vi "Rename Link.vi"(8 "error in (no error)":errorcluster, 9 "New Name":string, 10 "Old Name":string, 11 "Termination in":refnum<class "Termination.lvclass">) -> (0 "error out":errorcluster, 3 "Termination out":refnum<class "Termination.lvclass">)   [LabVIEW 2015, in "Termination.lvclass"]
uses:
  Termination.lvclass
  Termination.lvclass/Termination.ctl
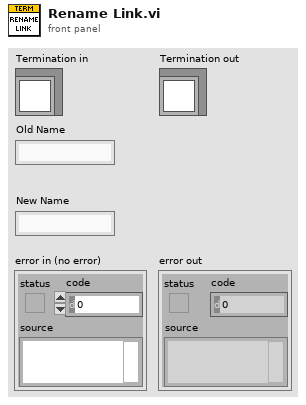
[diagram p1: front panel]
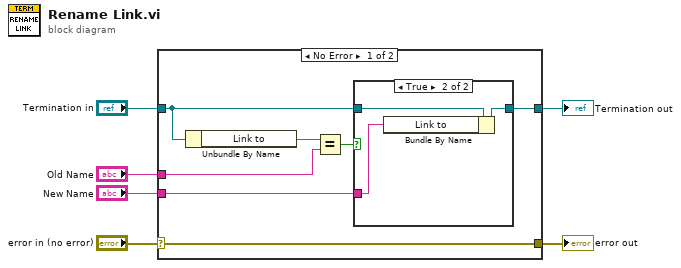
[diagram p0: block diagram]
diagram:
  n1 = case shown="No Error" "error in (no error)" {
    selector: "error in (no error)" -> [w13 w19]
    tunnel: [w13 w19] -> w5
    tunnel: [w9 w18] -> w3
    tunnel: "Termination in" -> [w10 w18]
    tunnel: "Old Name" -> [w11 _]
    tunnel: "New Name" -> [w7 _]
    frame No Error {
      n2 = Unbundle By Name(w10) -> ("Link to"=w12:string)
      n3 = Equal?(x=w12, y=w11) -> (x = y?=w8:bool)
      n4 = case shown="True" w8 {
        tunnel: w10 -> [w14 w17]
        tunnel: [w14 w16] -> w9
        tunnel: w7 -> [_ w15]
        frame False {
        }
        frame True {
          n5 = Bundle By Name(cluster=w17, "Link to"=w15) -> (w16:refnum<class "Termination.lvclass">)
        }
      }
    }
    frame Error {
    }
  }
  "error out" <- w5
  "Termination out" <- w3
